vi "Create New.vi"(8 "error in (no error)":errorcluster, 9 "Connection Timeout (10000 ms)":i32=10000, 10 "URL":string) -> (0 "error out":errorcluster, 3 "MJPEG Reader out":refnum<data-value>)   [LabVIEW 2015, in "MJPEG Reader.lvclass"]
doc: "Create a new MJPEG Reader for the URL specified."
uses:
  MJPEG Reader.lvclass
  MJPEG Reader.lvclass/MJPEG Reader.ctl
  <vilib>/regexp/Match Regular Expression.xnode
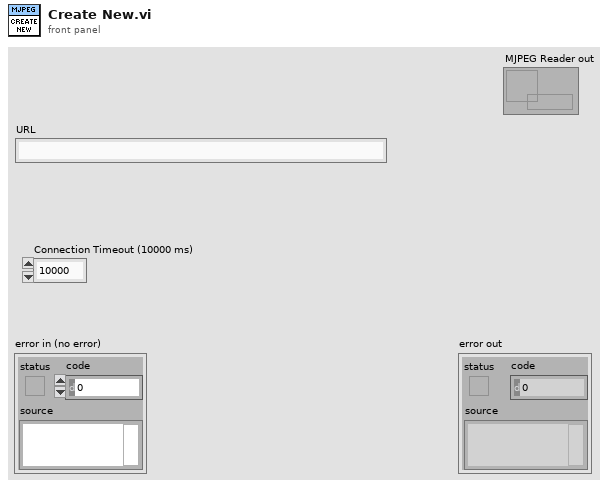
[diagram p1: front panel]
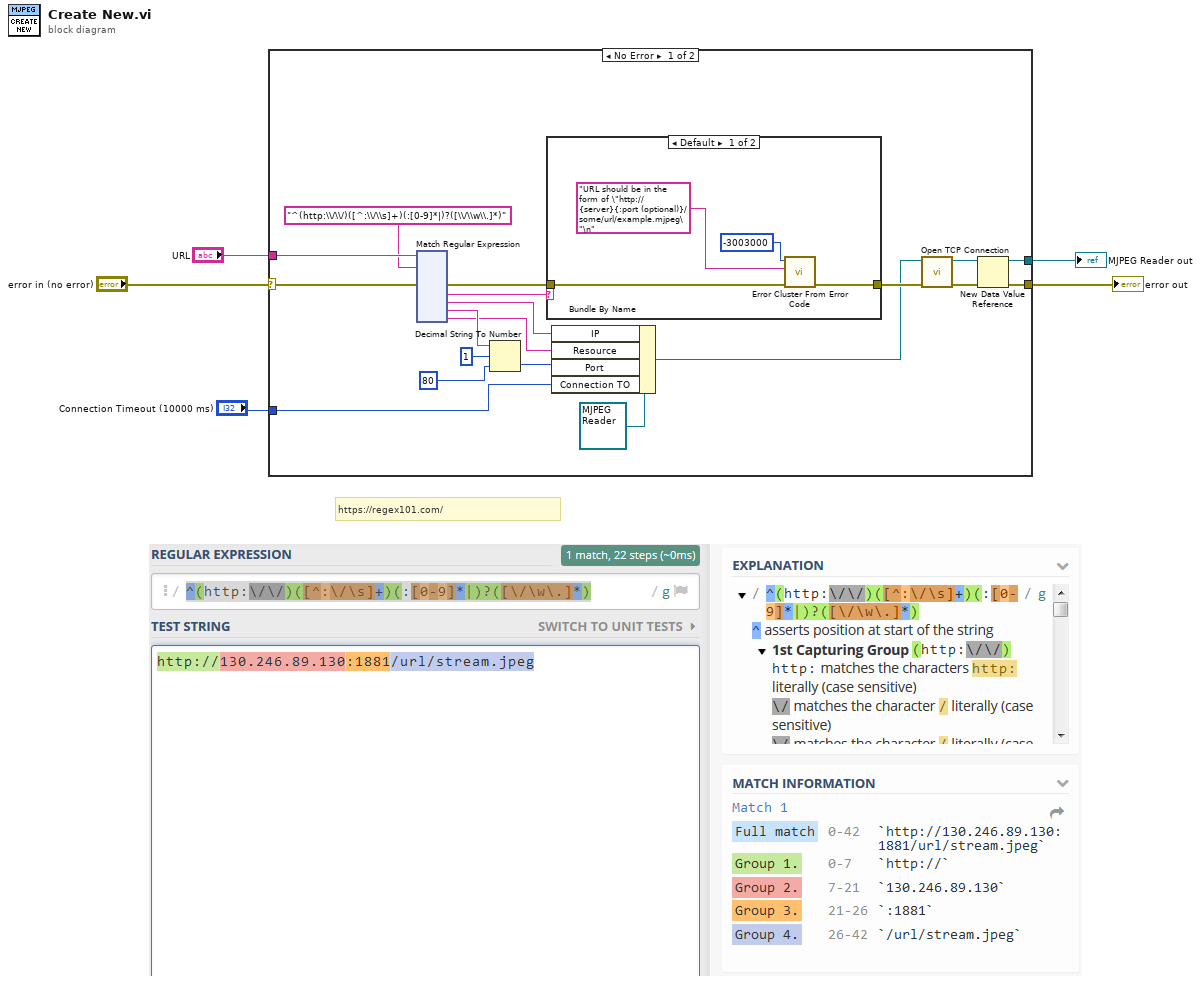
[diagram p0: block diagram]
diagram:
  # "https://regex101.com/"
  n1 = case shown="No Error" "error in (no error)" {
    selector: "error in (no error)" -> [w18 w149]
    tunnel: "URL" -> [w21 _]
    tunnel: [w9 w149] -> w3
    tunnel: [w10 _] -> w2
    tunnel: "Connection Timeout (10000 ms)" -> [w8 _]
    frame No Error {
      n2 = xnode "Match Regular Expression"("input string"=w21, "regular expression"="^(http:\\/\\/)([^:\\/\\s]+)(:[0-9]*|)?([\\/\\w\\.]*)", "error in"=w18) -> ("error out"=w13:errorcluster, "submatch 1"=w14:string, "submatch 2"=w19:string, "submatch 3"=w17:string, "submatch 4"=w16:string)  [unwired: 3 in, 4 out]
      n3 = Decimal String To Number(string=w17, offset=1, default (0L)=u16 80 ("default (0 I32)")) -> (number=w15:u16)  [unwired: 1 out]
      n4 = case shown="Default" w14 {
        tunnel: w13 -> [w28 w29]
        tunnel: [w27 w29] -> w12
        frame Default {
          n5 = call <vilib>:"Error Cluster From Error Code.vi"("error in (no error)"=w28, "error message (\"\")"="URL should be in the form of \"http://{server}{:port (optional)}/some/url/example.mjpeg\"\n" ("error message (\"\")"), "error code (0)"=-3003000) -> ("error out"=w27:errorcluster)  [unwired: 6 in]
        }
        frame "http://" {
        }
      }
      n6 = Bundle By Name(cluster=refnum<class "MJPEG Reader.lvclass"> refnum ("Scope Streamer Grabber in"), "IP"=w19, "Resource"=w16, "Port"=w15, "Connection TO"=w8) -> (w11:refnum<class "MJPEG Reader.lvclass">)
      n7 = call "Open TCP Connection.vi"("error in (no error)"=w12, "MJPEG Reader in"=w11) -> ("error out"=w6:errorcluster, "MJPEG Reader out"=w7:refnum<class "MJPEG Reader.lvclass">)  [unwired: 8 in]
      n8 = New Data Value Reference(data value=w7, error in=w6) -> (data value reference=w10:refnum<data-value>, error out=w9:errorcluster)
    }
    frame Error {
    }
  }
  "error out" <- w3
  "MJPEG Reader out" <- w2
